vi "Close.vi"(8 "error in (no error)":errorcluster, 11 "UDP in":refnum<class "UDP.lvclass">) -> (0 "error out":errorcluster, 3 "UDP out":refnum<class "UDP.lvclass">)   [LabVIEW 2018, in "UDP.lvclass"]
doc: "UDP.lvclass:Close.vi\n\nThis is the Close VI for the UDP class.\n\nInstrument Communication Module Version 1.0\nJanuary, 2017 Original Code Consulting David Thomson\n www.originalcode.com"
uses:
  UDP.lvclass
  UDP.lvclass/UDP.ctl
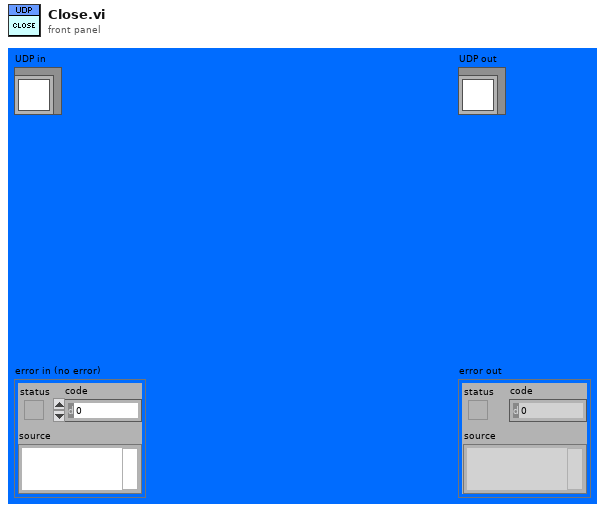
[diagram p1: front panel]
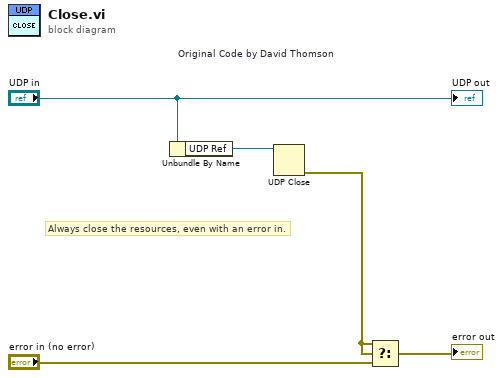
[diagram p0: block diagram]
diagram:
  # "Always close the resources, even with an error in."
  n1 = Unbundle By Name "Original Code by David Thomson"("UDP in") -> ("UDP Ref"=w4:refnum<k16>)
  n2 = UDP Close(connection ID=w4) -> (error out=w2:errorcluster)  [unwired: 1 in, 1 out]
  n3 = Select(t=w2, s=w2, f="error in (no error)") -> (s? t:f=→"error out":errorcluster)
  "UDP out" <- "UDP in"
